vi "HEWH MW100 Cut Unneeded Data.vi"(10 "MW100 Data In":string[][](array[string])) -> (2 "MW100 Data Out":string[][](array[string]))   [LabVIEW 2014]
panel:
  out "index of element 2":i32
  out "index of element":i32
  # "7"
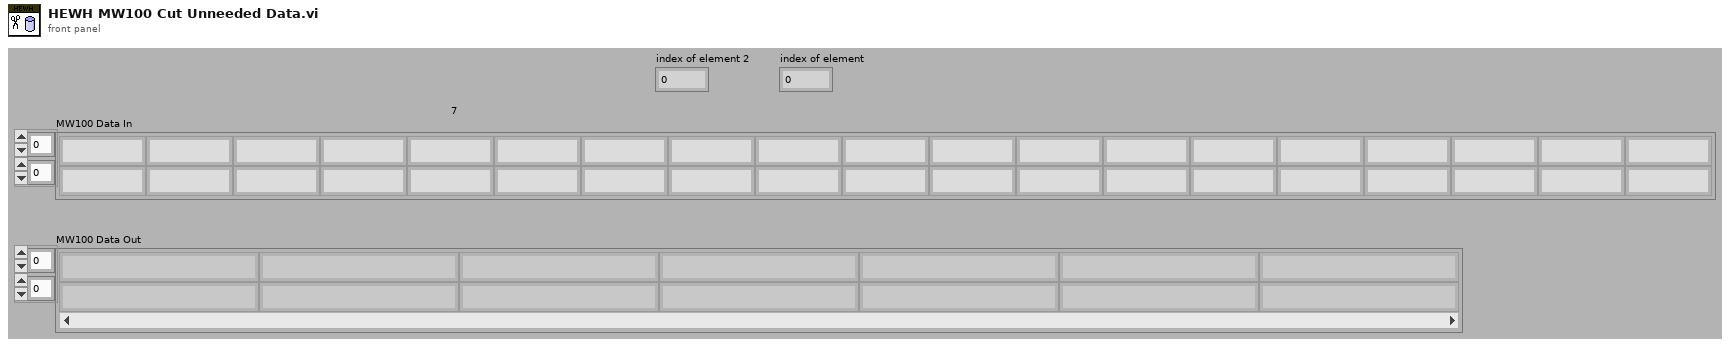
[diagram p1: front panel]
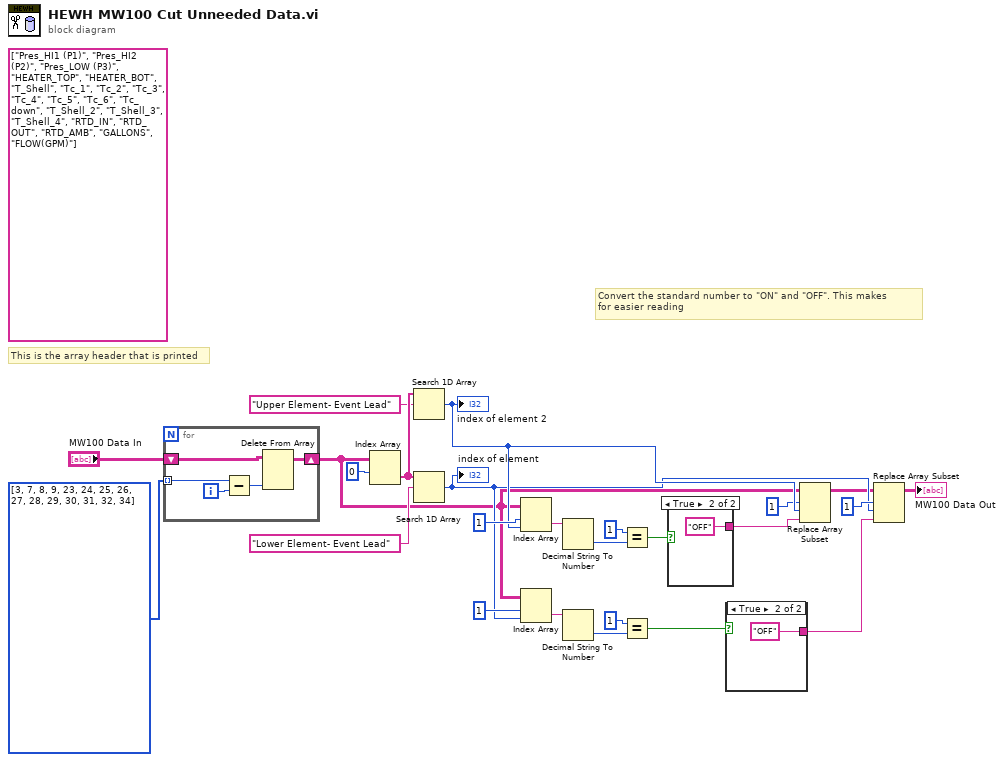
[diagram p0: block diagram]
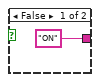
[diagram p2: hidden frame]
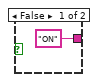
[diagram p3: hidden frame]
diagram:
  (unwired) string[] ["Pres_HI1 (P1)", "Pres_HI2 (P2)", "Pres_LOW (P3)", "HEATER_TOP", "HEATER_BOT", "T_Shell", "Tc_1", "Tc_2", "Tc_3", "Tc_4", "Tc_5", "Tc_6", "Tc_down", "T_Shell_2", "T_Shell_3", "T_Shell_4", "RTD_IN", "RTD_OUT", "RTD_AMB", "GALLONS", "FLOW(GPM)"] ("output array")
  # "Convert the standard number to \"ON\" and \"OFF\". This makes\nfor easier reading"
  # "This is the array header that is printed"
  n1 = for {
    tunnel: i32[] [3, 7, 8, 9, 23, 24, 25, 26, 27, 28, 29, 30, 31, 32, 34] ("Discarded MW100 Array Data") -> [w29] mode=indexing
    shift-right: [w27] -> w7
    shift-left: "MW100 Data In" -> [w26]
    i -> [w30]
    n2 = Subtract(x=w29, y=w30) -> (x-y=w28:i32)
    n3 = Delete From Array(array=w26, index (col)=w28) -> (array with subset deleted=w27:string[][])  [unwired: 2 in, 1 out]
  }
  n4 = Index Array(array=w7, index (row)=0) -> (element=w22:string[])  [unwired: 1 in]
  n5 = Search 1D Array(1D array=w22, element="Upper Element- Event Lead") -> (index of element=w16:i32)  [unwired: 1 in]
  "index of element 2" <- w16
  n6 = Search 1D Array(1D array=w22, element="Lower Element- Event Lead") -> (index of element=w10:i32)  [unwired: 1 in]
  "index of element" <- w10
  n7 = Index Array(array=w7, index (row)=1 ("disabled index (row)"), index (col)=w16) -> (element=w6:string)
  n8 = Index Array(array=w7, index (row)=1 ("disabled index (row)"), index (col)=w10) -> (element=w3:string)
  n9 = Decimal String To Number(string=w6) -> (number=w5:i32)  [unwired: 2 in, 1 out]
  n10 = Decimal String To Number(string=w3) -> (number=w2:i32)  [unwired: 2 in, 1 out]
  n11 = Equal?(x=1, y=w5) -> (x = y?=w17:bool)
  n12 = Equal?(x=1, y=w2) -> (x = y?=w13:bool)
  n13 = case shown="True" w17 {
    tunnel: ["ON" "OFF"] -> w14
    frame False {
    }
    frame True {
    }
  }
  n14 = case shown="True" w13 {
    tunnel: ["ON" "OFF"] -> w11
    frame False {
    }
    frame True {
    }
  }
  n15 = Replace Array Subset(array=w7, new element=w14, index (row)=1 ("disabled index (row)"), index (col)=w16) -> (w9:string[][])
  n16 = Replace Array Subset(array=w9, new element=w11, index (row)=1 ("disabled index (row)"), index (col)=w10) -> (→"MW100 Data Out":string[][])
